vi "Script_Create Steering Frame_by Type.vi"(8 "error in (no error)":errorcluster, 10 "owner diagram refnum":refnum<vi>, 11 "steering frame in":refnum<class "NI_Robotics_Steering Frame.lvclass">) -> (0 "error out":errorcluster, 1 "bundler input terminal refnums":refnum<vi>[](array[refnum]), 2 "steering frame out terminal refnum":refnum<vi>, 3 "steering frame out":refnum<class "NI_Robotics_Steering Frame.lvclass">, 4 "error out terminal refnum":refnum<vi>, 5 "wheels":refnum<class "NI_Robotics_Wheel.lvclass">[](array[class]), 6 "error in terminal refnum":refnum<vi>)   [LabVIEW 2017, in "NI_Robotics_Scripting Utilities.lvlib"]
uses:
  <vilib>/robotics/Utilities/Scripting/NI_Robotics_Scripting Utilities.lvlib
  <vilib>/robotics/Steering/Steering Frame/NI_Robotics_Steering Frame.lvclass
  <vilib>/robotics/Steering/Wheel/NI_Robotics_Wheel.lvclass
  <vilib>/robotics/Steering/Steering Frame/NI_Robotics_Steering Frame.lvclass/NI_Robotics_Steering Frame.ctl
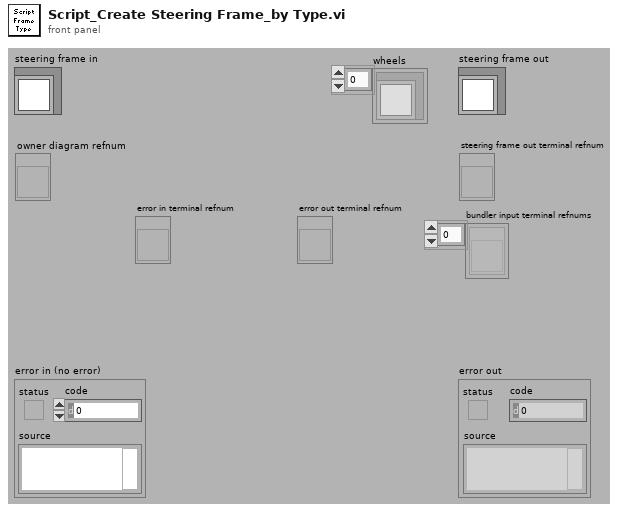
[diagram p1: front panel]
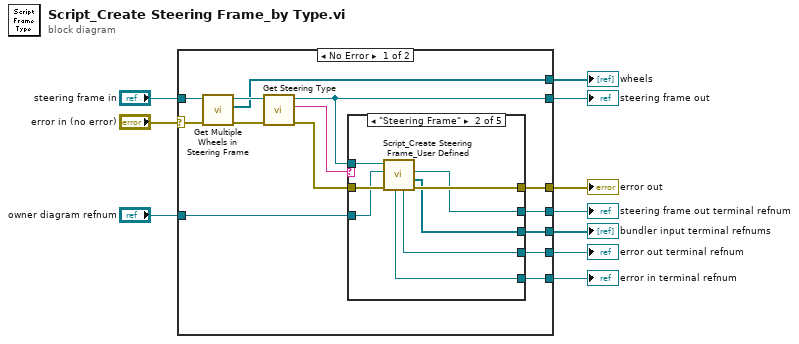
[diagram p0: block diagram]
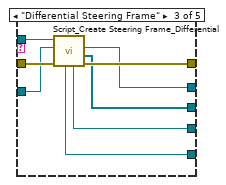
[diagram p3: hidden frame]
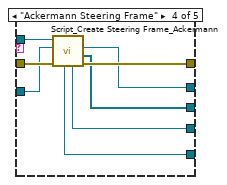
[diagram p4: hidden frame]
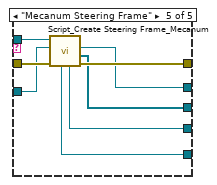
[diagram p5: hidden frame]
diagram:
  n1 = case shown="No Error" "error in (no error)" {
    selector: "error in (no error)" -> [w14 w58]
    tunnel: "steering frame in" -> [w16 w59]
    tunnel: [w11 w59] -> w8
    tunnel: [w22 w58] -> w7
    tunnel: "owner diagram refnum" -> [w21 _]
    tunnel: [w19 _] -> w1
    tunnel: [w17 _] -> w5
    tunnel: [w18 _] -> w4
    tunnel: [w12 _] -> w3
    tunnel: [w20 _] -> w2
    frame No Error {
      n2 = call <vilib>:"Get Multiple Wheels in Steering Frame.vi"("error in (no error)"=w14, "steering frame in"=w16) -> ("error out"=w13:errorcluster, "wheels"=w12:refnum<class "NI_Robotics_Wheel.lvclass">[], "steering frame out"=w15:refnum<class "NI_Robotics_Steering Frame.lvclass">)  [unwired: 3 in, 4 out]
      n3 = call-dynamic "Get Steering Type.vi"("error in (no error)"=w13, "steering frame in"=w15) -> ("error out"=w23:errorcluster, "steering type"=w24:string, "steering frame out"=w11:refnum<class "NI_Robotics_Steering Frame.lvclass">)  [unwired: 7 in]
      n4 = case shown="\"Steering Frame\"" w24 {
        tunnel: w11 -> [_ w33 w41 w49 w57]
        tunnel: w23 -> [w25 w32 w40 w48 w56]
        tunnel: [w25 w30 w38 w46 w54] -> w22
        tunnel: w21 -> [_ w31 w39 w47 w55]
        tunnel: [_ w29 w37 w45 w53] -> w20
        tunnel: [_ w28 w36 w44 w52] -> w19
        tunnel: [_ w27 w35 w43 w51] -> w18
        tunnel: [_ w26 w34 w42 w50] -> w17
        frame Default {
        }
        frame "Steering Frame" {
          n5 = call <vilib>:"Script_Create Steering Frame_User Defined.vi"("error in (no error)"=w32, "owner diagram refnum"=w31, "steering frame in"=w33) -> ("error out"=w30:errorcluster, "bundler input terminal refnums"=w28:refnum<vi>[], "steering frame out terminal refnum"=w29:refnum<vi>, "error out terminal refnum"=w27:refnum<vi>, "error in terminal refnum"=w26:refnum<vi>)  [unwired: 4 in]
        }
        frame "Differential Steering Frame" {
          n6 = call <vilib>:"Script_Create Steering Frame_Differential.vi"("error in (no error)"=w40, "owner diagram refnum"=w39, "steering frame in"=w41) -> ("error out"=w38:errorcluster, "bundler input terminal refnums"=w36:refnum<vi>[], "steering frame out terminal refnum"=w37:refnum<vi>, "error out terminal refnum"=w35:refnum<vi>, "error in terminal refnum"=w34:refnum<vi>)  [unwired: 4 in]
        }
        frame "Ackermann Steering Frame" {
          n7 = call <vilib>:"Script_Create Steering Frame_Ackermann.vi"("error in (no error)"=w48, "owner diagram refnum"=w47, "steering frame in"=w49) -> ("error out"=w46:errorcluster, "bundler input terminal refnums"=w44:refnum<vi>[], "steering frame out terminal refnum"=w45:refnum<vi>, "error out terminal refnum"=w43:refnum<vi>, "error in terminal refnum"=w42:refnum<vi>)  [unwired: 4 in]
        }
        frame "Mecanum Steering Frame" {
          n8 = call <vilib>:"Script_Create Steering Frame_Mecanum.vi"("error in (no error)"=w56, "owner diagram refnum"=w55, "steering frame in"=w57) -> ("error out"=w54:errorcluster, "bundler input terminal refnums"=w52:refnum<vi>[], "steering frame out terminal refnum"=w53:refnum<vi>, "error out terminal refnum"=w51:refnum<vi>, "error in terminal refnum"=w50:refnum<vi>)  [unwired: 4 in]
        }
      }
    }
    frame Error {
    }
  }
  "error out" <- w7
  "steering frame out" <- w8
  "steering frame out terminal refnum" <- w2
  "error out terminal refnum" <- w4
  "error in terminal refnum" <- w5
  "wheels" <- w3
  "bundler input terminal refnums" <- w1
